vi "Naming Check.vi"(8 "error in (no error)":errorcluster, 11 "Name(\"\" to use uuid)":string) -> (0 "error out":errorcluster, 3 "Name(dup)":string)   [LabVIEW 2020, in "Communicable State Machine.lvlib"]
uses:
  Communicable State Machine.lvlib
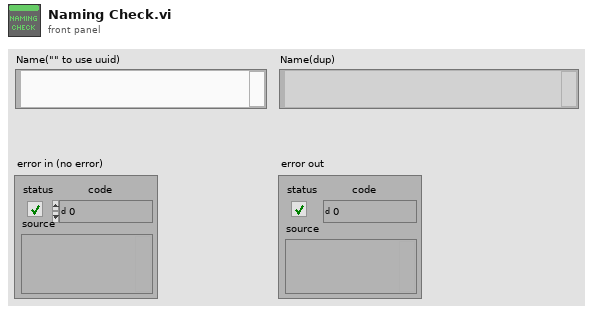
[diagram p1: front panel]
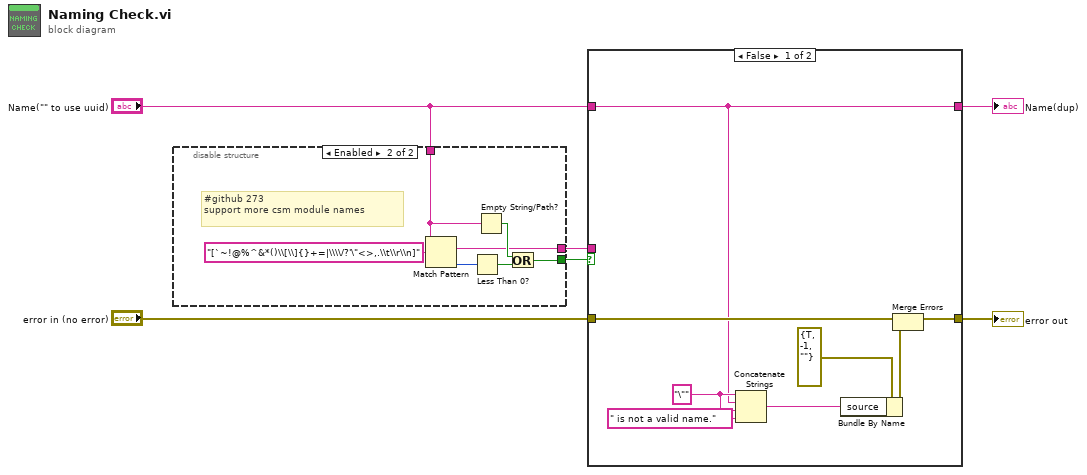
[diagram p0: block diagram]
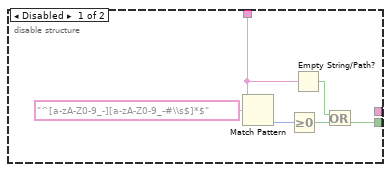
[diagram p2: hidden frame]
diagram:
  n1 = disable-structure shown="Enabled" {
    disable-tunnel: "Name(\"\" to use uuid)" -> [w9 w14]
    disable-tunnel: [w8 w15] -> w2
    disable-tunnel: [_ w13] -> w1
    frame Disabled {
      n2 = Match Pattern(string=w9, regular expression="^[a-zA-Z0-9_-][a-zA-Z0-9_-#\\s$]*$") -> (offset past match=w11:i32)  [unwired: 1 in, 3 out]
      n3 = Greater Or Equal To 0?(x=w11) -> (x >= 0?=w10:bool)
      n4 = Empty String/Path?(string/path=w9) -> (empty?=w7:bool)
      n5 = Or(x=w7, y=w10) -> (x .or. y?=w8:bool)
    }
    frame Enabled {
      # "#github 273 \nsupport more csm module names"
      n6 = Match Pattern(string=w14, regular expression="[`~!@%^&*()\\[\\]{}+=|\\\\/?'\"<>,.\\t\\r\\n]") -> (match substring=w13:string, offset past match=w18:i32)  [unwired: 1 in, 2 out]
      n7 = Less Than 0?(x=w18) -> (x < 0?=w17:bool)
      n8 = Empty String/Path?(string/path=w14) -> (empty?=w16:bool)
      n9 = Or(x=w16, y=w17) -> (x .or. y?=w15:bool)
    }
  }
  n10 = case shown="False" w2 {
    tunnel: "error in (no error)" -> [w27 w29]
    tunnel: [w26 w29] -> w5
    tunnel: [w23 w28] -> w4
    tunnel: "Name(\"\" to use uuid)" -> [w23 w28]
    tunnel: w1 -> [_ _]
    frame False {
      w24 = "\"" ("string")
      n11 = Concatenate Strings(w24, w23, w24, " is not a valid name." ("string")) -> (w20:string)
      n12 = Bundle By Name(cluster=errorcluster {"status"=TRUE, "code"=-1, "source"=""} ("error in"), "source"=w20) -> (w21:errorcluster)
      n13 = Merge Errors(w27, w21) -> (w26:errorcluster)
    }
    frame True {
    }
  }
  "error out" <- w5
  "Name(dup)" <- w4
